vi "Calculate Final Completion Times of Jobs.vi"(11 "Completion Times (MxJ)":i32[][](array[numeric])) -> (3 "Job Completion Times":i32[](array[numeric]))   [LabVIEW 2013, in "Scheduler.lvclass"]
uses:
  Scheduler.lvclass
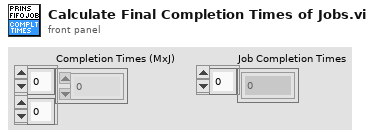
[diagram p1: front panel]
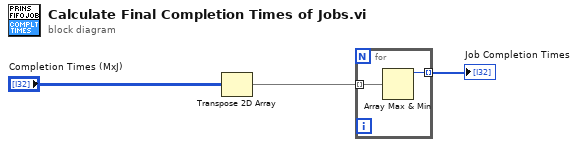
[diagram p0: block diagram]
diagram:
  n1 = Transpose 2D Array(2D array="Completion Times (MxJ)") -> (transposed array=w2:i32[][])
  n2 = for {
    tunnel: w2 -> [w5] mode=indexing
    tunnel: [w4] -> w1 mode=indexing
    n3 = Array Max & Min(array=w5) -> (max value=w4:i32)  [unwired: 3 out]
  }
  "Job Completion Times" <- w1
